vi "Jacobi Iteration (abs residual).vi"(4 "max. iters":i32=10000, 5 "abs. tol":dbl=1e-05, 6 "B":dbl[](array[numeric])=[6.0, 25.0, -11.0, 15.0], 7 "A":dbl[][](array[numeric])=[[10.0, -1.0, 2.0, 0.0], [-1.0, 11.0, -1.0, 3.0], [2.0, -1.0, 10.0, -1.0], [0.0, 3.0, -1.0, 8.0]]) -> (0 "Converged?":bool=TRUE, 1 "Iterations":i32=24, 3 "X":dbl[](array[numeric])=[1.0000000008366592, 1.9999999985888712, -0.9999999989100756, 0.9999999984529894])   [LabVIEW 2017]
uses:
  <vilib>/Analysis/baseanly.llb/A x Vector.vi
  <vilib>/Analysis/NI_AALBase.lvlib
panel:
  in  "Stop":bool
  out "Residual":sgl(graph)
  # "PN 21/10/17"
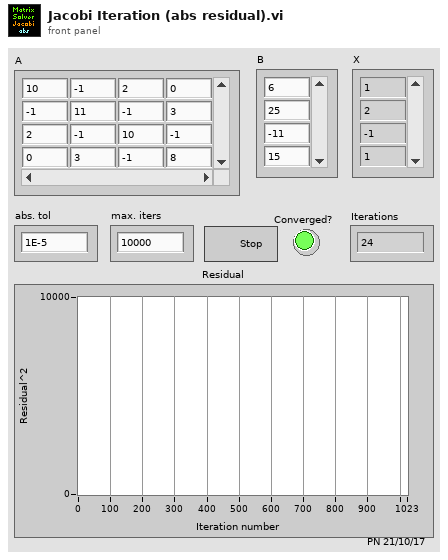
[diagram p1: front panel]
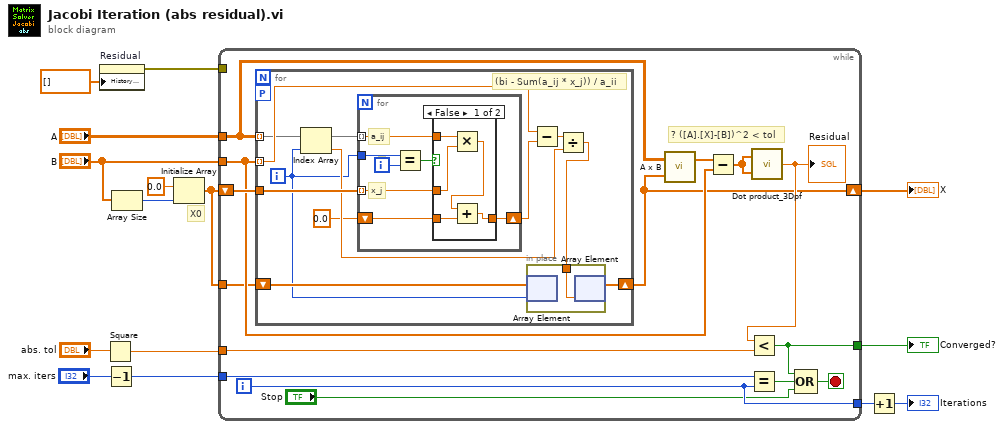
[diagram p0: block diagram]
diagram:
  # "X0"
  n1 = property on="Residual" class="WFChart (strict)"("History Data"=sgl[] []) -> (error out=w3:errorcluster)  [unwired: 2 in, 1 out]
  n2 = Square(x="abs. tol") -> (x^2=w4:dbl)
  n3 = Decrement(x="max. iters") -> (x-1=w11:i32)
  n4 = Array Size(array="B") -> (size(s)=w14:i32)
  n5 = Initialize Array(0.0 ("element"), w14) -> (w2:dbl[])
  n6 = while {
    tunnel: "A" -> [w26]
    tunnel: "B" -> [w24]
    tunnel: w4 -> [w23]
    shift-right: [w19] -> w7
    shift-left: w2 -> [w30]
    tunnel: w11 -> [w28]
    tunnel: [w27] -> w10
    tunnel: [w16] -> w1
    tunnel: w3 -> [_]
    tunnel: w2 -> [w20]
    i -> [w27]
    stop <- w29 stop-if-true
    # "? ([A].[X]-[B])^2 < tol"
    n7 = for {
      tunnel: w24 -> [w40] mode=indexing
      tunnel: w26 -> [w37] mode=indexing
      tunnel: w30 -> [w41]
      workers-P: _ -> [_]
      shift-right: [w33] -> w19
      shift-left: w20 -> [w34]
      i -> [w31]
      # "(bi - Sum(a_ij * x_j)) / a_ii"
      n8 = Index Array(array=w37, index=w31) -> (element=w38:dbl)
      n9 = for {
        tunnel: w31 -> [w48]
        tunnel: w37 -> [w46] mode=indexing
        tunnel: w41 -> [w45] mode=indexing
        shift-right: [w44] -> w35
        shift-left: 0.0 ("element") -> [w43]
        i -> [w49]
        # "x_j"
        # "a_ij"
        # "j"
        n10 = Equal?(x=w48, y=w49) -> (x = y?=w47:bool)
        n11 = case shown="False" w47 {
          tunnel: w46 -> [w54 _]
          tunnel: w45 -> [w53 _]
          tunnel: [w51 w55] -> w44
          tunnel: w43 -> [w52 w55]
          frame False {
            n12 = Multiply(x=w54, y=w53) -> (x*y=w50:dbl)
            n13 = Add(x=w50, y=w52) -> (x+y=w51:dbl)
          }
          frame True {
          }
        }
      }
      n14 = Subtract(x=w40, y=w35) -> (x-y=w39:dbl)
      n15 = Divide(x=w39, y=w38) -> (x/y=w32:dbl)
      n16 = in-place {
        in-place-border: w32 -> [w42]
        n17 = in-place-array #1(w34, w31) -> ()  [unwired: 1 out]
        n18 = in-place-array #1(w42) -> (w33:dbl[])  [unwired: 1 out]
      }
    }
    n19 = call-poly <vilib>:"A x B.vi"("Vector"=w19, "A"=w26) -> ("A x Vector"=w25:dbl[])  [unwired: 1 out]
    n20 = Subtract(x=w25, y=w24) -> (x-y=w22:dbl[])
    n21 = Equal?(x=w28, y=w27) -> (x = y?=w18:bool)
    n22 = call "Dot product_3Dpf.vi"("B"=w22, "A"=w22) -> ("A . B"=w21:sgl)
    "Residual" <- w21
    n23 = Less?(x=w21, y=w23) -> (x < y?=w16:bool)
    n24 = Compound Arithmetic op=OR(w16, w18, "Stop") -> (w29:bool)
  }
  "X" <- w7
  "Converged?" <- w1
  n25 = Increment(x=w10) -> (x+1=→"Iterations":i32)
